vi "addObjectIDElement.vi"(6 "Add to Front of Object (true)":bool=TRUE, 7 "Name":string, 8 "error in (no error)":errorcluster, 9 "Value":string, 10 "Replace? (false)":bool, 11 "tBSONDocument in":refnum<class "tBSONDocument.lvclass">) -> (0 "error out":errorcluster, 3 "tBSONDocument out":refnum<class "tBSONDocument.lvclass">)   [LabVIEW 2013, in "BSON.lvlib" / "tBSONDocument.lvclass"]
doc: "Adds an Object ID to a BSON document."
uses:
  tBSONDocument.lvclass
  BSONElements/tBSONObjectID/tBSONObjectID.lvclass
  tBSONElement/tBSONElement.lvclass
  tBSONElement/setName.vi
  BSONElements/tBSONObjectID/setValue.vi
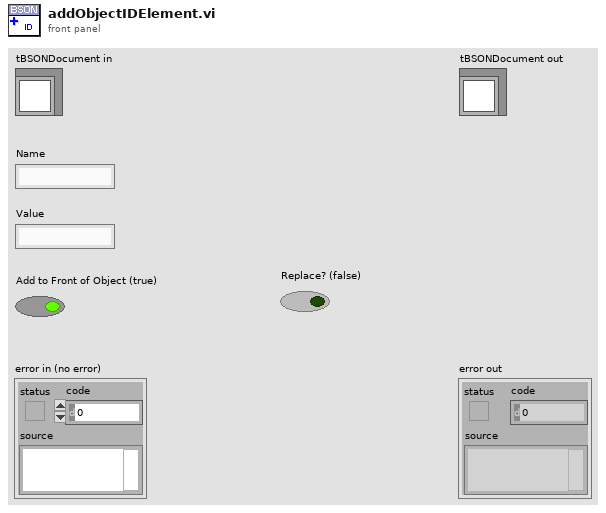
[diagram p1: front panel]
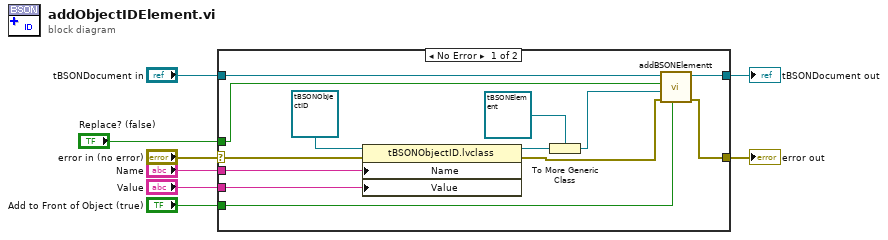
[diagram p0: block diagram]
diagram:
  n1 = case shown="No Error" "error in (no error)" {
    selector: "error in (no error)" -> [w20 w23]
    tunnel: [w11 w23] -> w7
    tunnel: [w13 w22] -> w5
    tunnel: "tBSONDocument in" -> [w14 w22]
    tunnel: "Name" -> [w19 _]
    tunnel: "Value" -> [w18 _]
    tunnel: "Add to Front of Object (true)" -> [w10 _]
    tunnel: "Replace? (false)" -> [w9 _]
    frame No Error {
      n2 = property class="tBSONObjectID.lvclass"(reference=refnum<class "tBSONObjectID.lvclass"> refnum ("BSON.lvlib:tBSONObjectID.lvclass"), error in=w20, "Name"=w19, "Value"=w18) -> (reference out=w17:refnum<class "tBSONObjectID.lvclass">, error out=w12:errorcluster)
      n3 = To More Generic Class(target class=refnum<class "tBSONElement.lvclass"> refnum ("BSON.lvlib:tBSONElement.lvclass"), reference=w17) -> (generic class reference=w15:refnum<class "tBSONElement.lvclass">)
      n4 = call "addBSONElementt.vi"("Add to front of object (false)"=w10, "error in (no error)"=w12, "Element"=w15, "Replace? (false)"=w9, "tBSONDocument in"=w14) -> ("error out"=w11:errorcluster, "tBSONDocument out"=w13:refnum<class "tBSONDocument.lvclass">)  [unwired: 5 in]
    }
    frame Error {
    }
  }
  "error out" <- w7
  "tBSONDocument out" <- w5
